vi "lab2_1.vi"() -> ()   [LabVIEW 2026]
uses:
  <vilib>/numeric/Random Number (Range) DBL.vi
panel:
  out "x-y":u32
  out "millisecond timer value 2":u32
  out "millisecond timer value":u32
  out "Number of tries":i32
  out "x = y?":bool
  in  "Number to find":dbl
  out "number":dbl
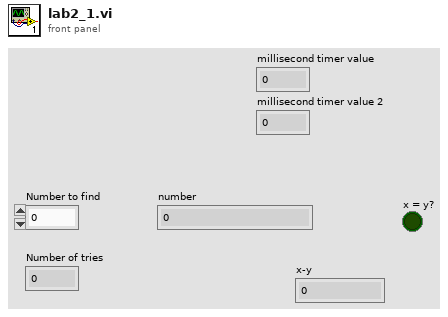
[diagram p1: front panel]
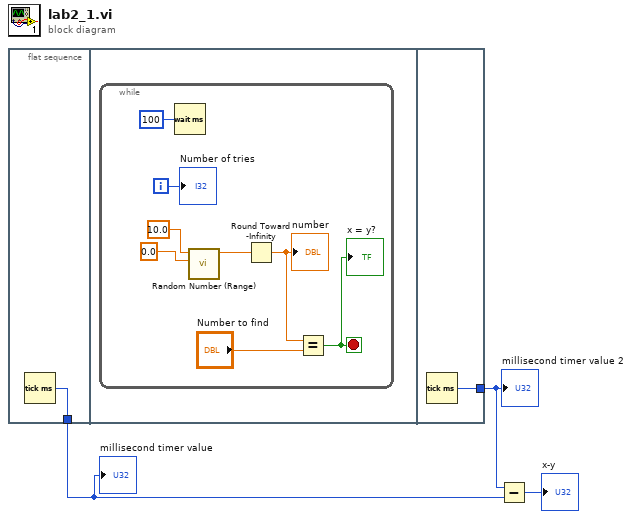
[diagram p0: block diagram]
diagram:
  n1 = flat-sequence {
    tunnel: [w4] -> w1
    tunnel: [w13] -> w2
    frame #0 {
      n2 = Tick Count (ms)() -> (millisecond timer value=w4:u32)
    }
    frame #1 {
      n3 = while {
        i -> [w6]
        stop <- w7 stop-if-true
        n4 = Wait (ms)(milliseconds to wait=u32 100) -> ()  [unwired: 1 out]
        n5 = call-poly <vilib>:"Random Number (Range).vi"("lower bound (0)"=0.0, "upper bound (100)"=10.0) -> ("number"=w10:dbl)  [unwired: 9 in]
        n6 = Round Toward -Infinity(1:w10) -> (0:w8:dbl)
        "number" <- w8
        n7 = Equal?(x=w8, y="Number to find") -> (x = y?=w7:bool)
        "x = y?" <- w7
        "Number of tries" <- w6
      }
    }
    frame #2 {
      n8 = Tick Count (ms)() -> (millisecond timer value=w13:u32)
    }
  }
  n9 = Subtract(x=w2, y=w1) -> (x-y=→"x-y":u32)
  "millisecond timer value" <- w1
  "millisecond timer value 2" <- w2
